vi "Configure Delta Computation.vi"(7 "Wire Unit (0: Sigma A)":i32(ring) items=["Sigma A", "Sigma B", "Sigma C"], 8 "error in (no error)":errorcluster, 9 "Delta Measure Mode (0: rms)":i32(ring) items=["rms", "mean", "dc", "r-mean", "ac"], 10 "Delta Measure Type (1: Difference)":i32(ring)=1 items=["Difference"=1, "3P3W > 3V3A"=2, "Star > Delta"=3, "Delta > Star"=4], 11 "VISA resource name":refnum<visa-resource-name>) -> (0 "error out":errorcluster, 3 "VISA resource name out":refnum<visa-resource-name>)   [LabVIEW 2021, in "Yokogawa WT1800 Series.lvlib"]
doc: "The sum or difference of the instantaneous voltage or current values (sampled data) between the elements in a wiring unit can be used to determine various types of data such as the differential voltage and phase voltage.\n\n<b>Note:</b>\nThis setting valid on models with the delta computation (/DT) option."
uses:
  <instrlib>/Yokogawa WT1800 Series/Yokogawa WT1800 Series.lvlib
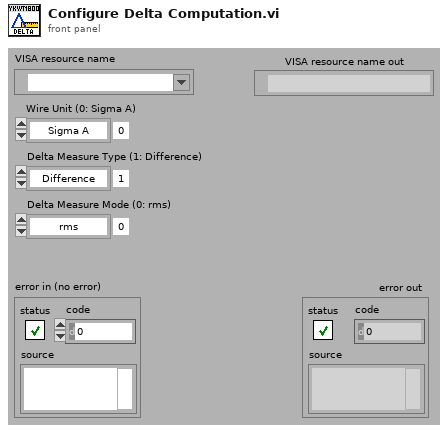
[diagram p1: front panel]
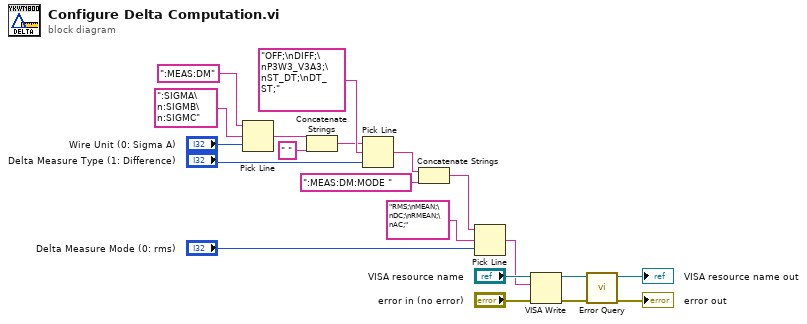
[diagram p0: block diagram]
diagram:
  n1 = Pick Line ("ライン選択")(string ("")=":MEAS:DM", multi-line string=":SIGMA\n:SIGMB\n:SIGMC" ("複数行文字列"), line index="Wire Unit (0: Sigma A)") -> (output string=w8:string)
  n2 = Concatenate Strings(w8, " " ("文字列")) -> (w7:string)
  n3 = Pick Line ("ライン選択")(string ("")=w7, multi-line string="OFF;\nDIFF;\nP3W3_V3A3;\nST_DT;\nDT_ST;" ("複数行文字列"), line index="Delta Measure Type (1: Difference)") -> (output string=w3:string)
  n4 = Concatenate Strings(w3, ":MEAS:DM:MODE " ("文字列")) -> (w4:string)
  n5 = Pick Line ("ライン選択")(string ("")=w4, multi-line string="RMS;\nMEAN;\nDC;\nRMEAN;\nAC;" ("複数行文字列"), line index="Delta Measure Mode (0: rms)") -> (output string=w1:string)
  n6 = VISA Write ("VISA書き込み")(VISA resource name="VISA resource name", write buffer=w1, error in (no error)="error in (no error)") -> (VISA resource name out=w20:refnum<visa-resource-name>, error out=w19:errorcluster)  [unwired: 1 out]
  n7 = call <instrlib>:"Error Query.vi"("error in (no error)"=w19, "VISA resource name"=w20) -> ("error out"=→"error out":errorcluster, "VISA resource name out"=→"VISA resource name out":refnum<visa-resource-name>)  [unwired: 6 in, 2 out]
